vi "mitutoyo.vi"() -> ()   [LabVIEW 2015]
uses:
  <vilib>/Analysis/baseanly.llb/Mean (DBL).vi
  Global_mitu.vi
  <vilib>/Analysis/NI_AALBase.lvlib
panel:
  out "element":i32
  out "max value":dbl
  out "min value":dbl
  in  "DONE?":bool
  out "standard deviation":dbl format="%0.2f"
  out "mean":dbl format="%0.2f"
  out "Foil Name":string
  out "Output File path":path
  out "Result 9":bool
  out "Result 8":bool
  out "Result 7":bool
  out "Result 6":bool
  out "Result 5":bool
  out "Result 4":bool
  out "Result 3":bool
  out "Result 2":bool
  out "Result 1":bool
  in  "Open DataBase":bool
  out "9":bool
  out "8":bool
  out "7":bool
  out "6":bool
  out "5":bool
  out "4":bool
  out "3":bool
  out "2":bool
  out "1":bool
  in  "Table Control":string[][](table)
  in  "Stop\nMeasurement":bool
  # "Mitutoyo Honeycomb Measurements"
  # "Results"
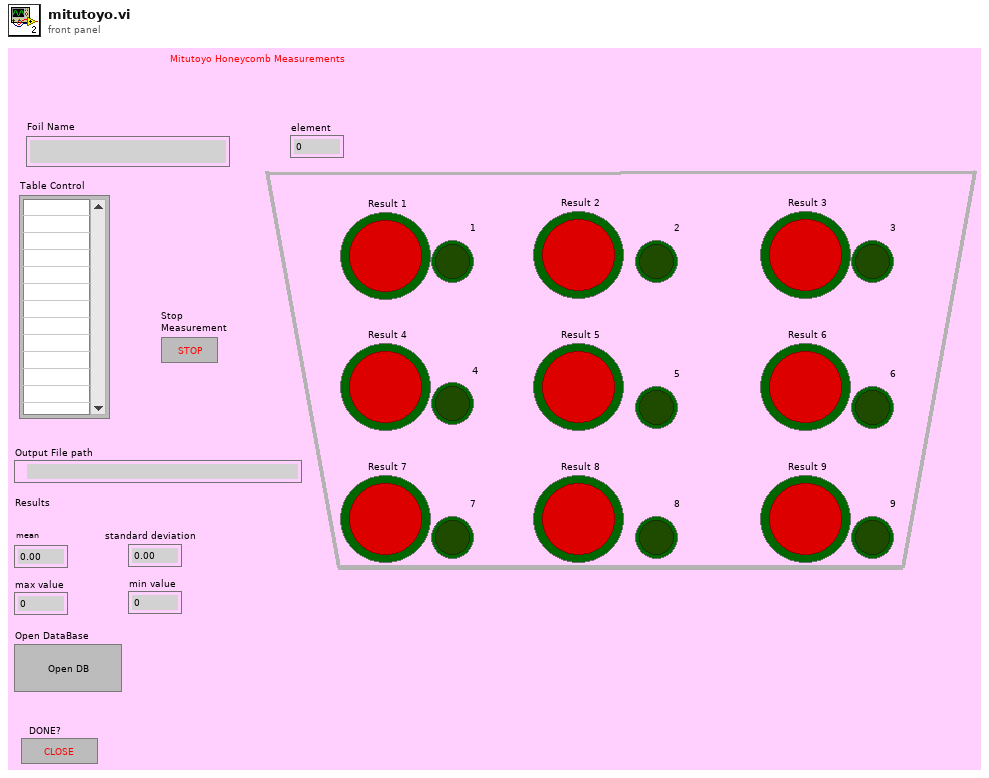
[diagram p1: front panel]
types:
  T1 = enum8{"Enabled", "Disabled", "Disabled and Grayed Out"}
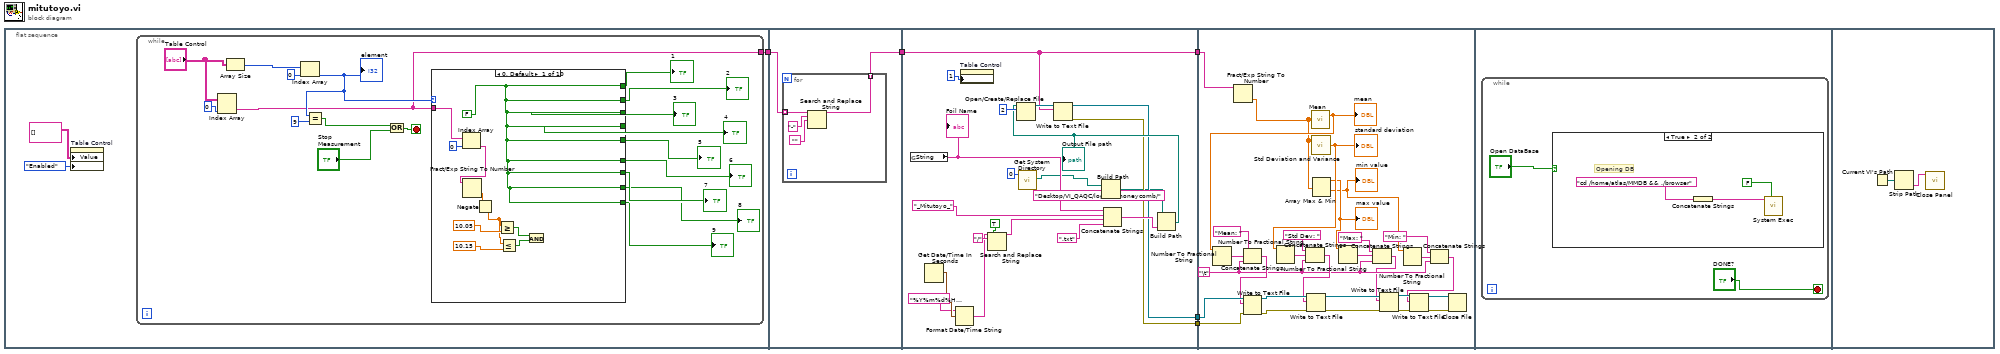
[diagram p0: block diagram]
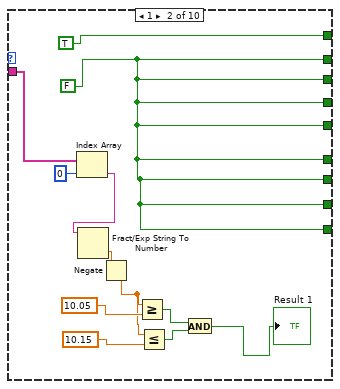
[diagram p2: hidden frame]
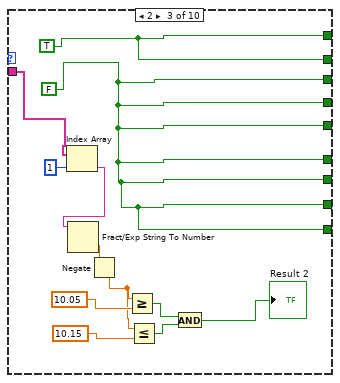
[diagram p3: hidden frame]
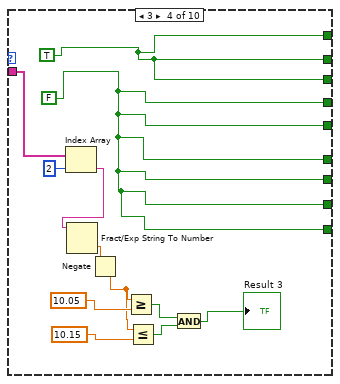
[diagram p4: hidden frame]
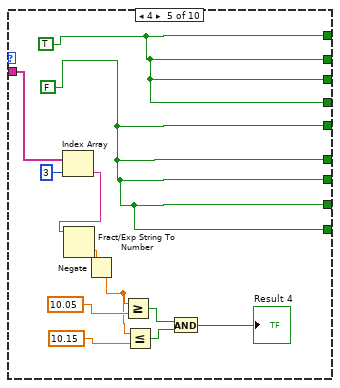
[diagram p5: hidden frame]
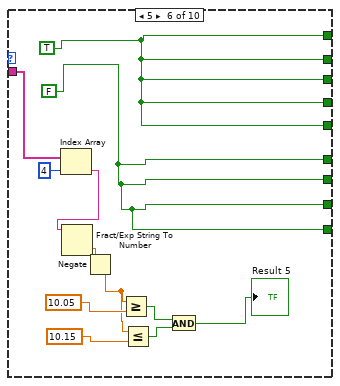
[diagram p6: hidden frame]
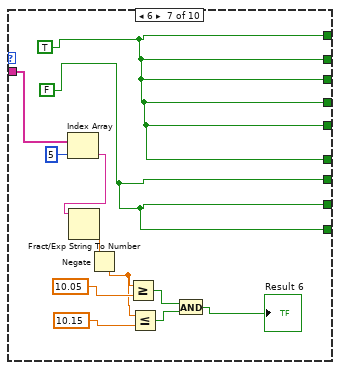
[diagram p7: hidden frame]
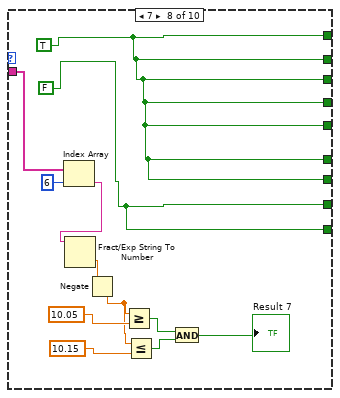
[diagram p8: hidden frame]
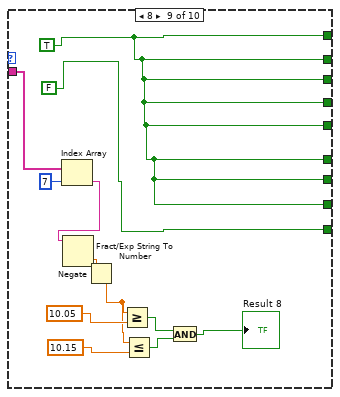
[diagram p9: hidden frame]
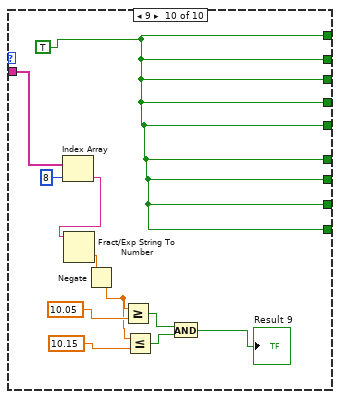
[diagram p10: hidden frame]
diagram:
  n1 = flat-sequence {
    tunnel: [w8] -> w2
    tunnel: w2 -> [w146]
    tunnel: [w145] -> w1
    tunnel: w1 -> [w151]
    tunnel: [w151] -> w5
    tunnel: [w160] -> w4
    tunnel: [w161] -> w3
    tunnel: w5 -> [w200]
    tunnel: w4 -> [w199]
    tunnel: w3 -> [w194]
    frame #0 {
      n2 = property on="Table Control" class="Tbl (strict)"("Value"=string[][] [] ("Table Control"), "DisabledEnum"=T1."Enabled" ("Disabled")) -> ()  [unwired: 2 in, 2 out]
      n3 = while {
        tunnel: [w10] -> w8
        stop <- w9 stop-if-true
        n4 = Index Array(array="Table Control", index (col)=0 ("index (row)")) -> (element=w10:string[])  [unwired: 1 in]
        n5 = Array Size(array="Table Control") -> (size(s)=w27:i32[])
        n6 = Index Array(array=w27, index=0) -> (element=w14:i32)
        "element" <- w14
        n7 = Equal?(x=w14, y=9) -> (x = y?=w11:bool)
        n8 = Or(x=w11, y="Stop\nMeasurement") -> (x .or. y?=w9:bool)
        n9 = case shown="0, Default" w14 {
          tunnel: [w37 TRUE w60 w73 w85 w97 w109 w121 w133 w144] -> w23
          tunnel: [w37 w48 w60 w73 w85 w97 w109 w121 w133 w144] -> w22
          tunnel: [w37 w48 w61 w73 w85 w97 w109 w121 w133 w144] -> w21
          tunnel: [w37 w48 w61 w72 w85 w97 w109 w121 w133 w144] -> w20
          tunnel: [w37 w48 w61 w72 w84 w97 w109 w121 w133 w144] -> w19
          tunnel: [w37 w48 w61 w72 w84 w96 w109 w121 w133 w144] -> w18
          tunnel: [w37 w48 w61 w72 w84 w96 w108 w121 w133 w144] -> w17
          tunnel: [w37 w48 w61 w72 w84 w96 w108 w120 w133 w144] -> w16
          tunnel: [w37 w48 w61 w72 w84 w96 w108 w120 FALSE w144] -> w15
          tunnel: w10 -> [w36 w40 w52 w64 w76 w88 w100 w112 w124 w136]
          frame 0, Default {
            w37 = FALSE
            n10 = Index Array(array=w36, index=0) -> (element=w34:string)
            n11 = Fract/Exp String To Number(string=w34) -> (number=w33:dbl)  [unwired: 3 in, 1 out]
            n12 = Negate(x=w33) -> (-x=w28:dbl)
            n13 = Greater Or Equal?(x=w28, y=10.05) -> (x >= y?=w32:bool)
            n14 = Less Or Equal?(x=w28, y=10.15) -> (x <= y?=w31:bool)
            n15 = And(x=w32, y=w31) -> ()  [unwired: 1 out]
          }
          frame 1 {
            w48 = FALSE
            n16 = Index Array(array=w40, index=0) -> (element=w41:string)
            n17 = Fract/Exp String To Number(string=w41) -> (number=w46:dbl)  [unwired: 3 in, 1 out]
            n18 = Negate(x=w46) -> (-x=w38:dbl)
            n19 = Greater Or Equal?(x=w38, y=10.05) -> (x >= y?=w45:bool)
            n20 = Less Or Equal?(x=w38, y=10.15) -> (x <= y?=w44:bool)
            n21 = And(x=w45, y=w44) -> (x .and. y?=→"Result 1":bool)
          }
          frame 2 {
            w61 = FALSE
            w60 = TRUE
            n22 = Index Array(array=w52, index=1) -> (element=w58:string)
            n23 = Fract/Exp String To Number(string=w58) -> (number=w57:dbl)  [unwired: 3 in, 1 out]
            n24 = Negate(x=w57) -> (-x=w50:dbl)
            n25 = Greater Or Equal?(x=w50, y=10.05) -> (x >= y?=w56:bool)
            n26 = Less Or Equal?(x=w50, y=10.15) -> (x <= y?=w55:bool)
            n27 = And(x=w56, y=w55) -> (x .and. y?=→"Result 2":bool)
          }
          frame 3 {
            w72 = FALSE
            w73 = TRUE
            n28 = Index Array(array=w64, index=2) -> (element=w70:string)
            n29 = Fract/Exp String To Number(string=w70) -> (number=w69:dbl)  [unwired: 3 in, 1 out]
            n30 = Negate(x=w69) -> (-x=w62:dbl)
            n31 = Greater Or Equal?(x=w62, y=10.05) -> (x >= y?=w68:bool)
            n32 = Less Or Equal?(x=w62, y=10.15) -> (x <= y?=w67:bool)
            n33 = And(x=w68, y=w67) -> (x .and. y?=→"Result 3":bool)
          }
          frame 4 {
            w84 = FALSE
            w85 = TRUE
            n34 = Index Array(array=w76, index=3) -> (element=w82:string)
            n35 = Fract/Exp String To Number(string=w82) -> (number=w81:dbl)  [unwired: 3 in, 1 out]
            n36 = Negate(x=w81) -> (-x=w74:dbl)
            n37 = Greater Or Equal?(x=w74, y=10.05) -> (x >= y?=w80:bool)
            n38 = Less Or Equal?(x=w74, y=10.15) -> (x <= y?=w79:bool)
            n39 = And(x=w80, y=w79) -> (x .and. y?=→"Result 4":bool)
          }
          frame 5 {
            w96 = FALSE
            w97 = TRUE
            n40 = Index Array(array=w88, index=4) -> (element=w94:string)
            n41 = Fract/Exp String To Number(string=w94) -> (number=w93:dbl)  [unwired: 3 in, 1 out]
            n42 = Negate(x=w93) -> (-x=w86:dbl)
            n43 = Greater Or Equal?(x=w86, y=10.05) -> (x >= y?=w92:bool)
            n44 = Less Or Equal?(x=w86, y=10.15) -> (x <= y?=w91:bool)
            n45 = And(x=w92, y=w91) -> (x .and. y?=→"Result 5":bool)
          }
          frame 6 {
            w108 = FALSE
            w109 = TRUE
            n46 = Index Array(array=w100, index=5) -> (element=w102:string)
            n47 = Fract/Exp String To Number(string=w102) -> (number=w103:dbl)  [unwired: 3 in, 1 out]
            n48 = Negate(x=w103) -> (-x=w98:dbl)
            n49 = Greater Or Equal?(x=w98, y=10.05) -> (x >= y?=w104:bool)
            n50 = Less Or Equal?(x=w98, y=10.15) -> (x <= y?=w105:bool)
            n51 = And(x=w104, y=w105) -> (x .and. y?=→"Result 6":bool)
          }
          frame 7 {
            w120 = FALSE
            w121 = TRUE
            n52 = Index Array(array=w112, index=6) -> (element=w118:string)
            n53 = Fract/Exp String To Number(string=w118) -> (number=w117:dbl)  [unwired: 3 in, 1 out]
            n54 = Negate(x=w117) -> (-x=w110:dbl)
            n55 = Greater Or Equal?(x=w110, y=10.05) -> (x >= y?=w116:bool)
            n56 = Less Or Equal?(x=w110, y=10.15) -> (x <= y?=w115:bool)
            n57 = And(x=w116, y=w115) -> (x .and. y?=→"Result 7":bool)
          }
          frame 8 {
            w133 = TRUE
            n58 = Index Array(array=w124, index=7) -> (element=w130:string)
            n59 = Fract/Exp String To Number(string=w130) -> (number=w129:dbl)  [unwired: 3 in, 1 out]
            n60 = Negate(x=w129) -> (-x=w122:dbl)
            n61 = Greater Or Equal?(x=w122, y=10.05) -> (x >= y?=w128:bool)
            n62 = Less Or Equal?(x=w122, y=10.15) -> (x <= y?=w127:bool)
            n63 = And(x=w128, y=w127) -> (x .and. y?=→"Result 8":bool)
          }
          frame 9 {
            w144 = TRUE
            n64 = Index Array(array=w136, index=8) -> (element=w142:string)
            n65 = Fract/Exp String To Number(string=w142) -> (number=w141:dbl)  [unwired: 3 in, 1 out]
            n66 = Negate(x=w141) -> (-x=w134:dbl)
            n67 = Greater Or Equal?(x=w134, y=10.05) -> (x >= y?=w140:bool)
            n68 = Less Or Equal?(x=w134, y=10.15) -> (x <= y?=w139:bool)
            n69 = And(x=w140, y=w139) -> (x .and. y?=→"Result 9":bool)
          }
        }
        "1" <- w23
        "2" <- w22
        "3" <- w21
        "4" <- w20
        "5" <- w19
        "6" <- w18
        "7" <- w17
        "8" <- w16
        "9" <- w15
      }
    }
    frame #1 {
      n70 = for {
        tunnel: w146 -> [w150] mode=indexing
        tunnel: [w147] -> w145 mode=indexing
        n71 = Search and Replace String(input string=w150, search string="-", replace string="") -> (result string=w147:string)  [unwired: 5 in, 3 out]
      }
    }
    frame #2 {
      n72 = global read "Global_mitu.vi" "String"() -> (w168:string)
      "Foil Name" <- w168
      n73 = Get Date/Time In Seconds() -> (seconds since 1Jan1904=w159:timestamp)
      n74 = Format Date/Time String(time format string (%c)="%Y%m%d%H%M", seconds (now)=w159) -> (date/time string=w157:string)  [unwired: 1 in]
      n75 = property on="Table Control" class="Tbl (strict)"("DisabledEnum"=1) -> ()  [unwired: 2 in, 2 out]
      n76 = Search and Replace String(replace all?=TRUE ("replace all? (F)"), input string=w157, search string="/") -> (result string=w166:string)  [unwired: 5 in, 3 out]
      n77 = call <vilib>:"Get System Directory.vi"("system directory type"=0) -> ("system directory"=w154:path)  [unwired: 10 in]
      n78 = Build Path(base path=w154, name or relative path="Desktop/VI_QAQC/logfiles/honeycomb/") -> (appended path=w153:path)
      n79 = Concatenate Strings(w168, "_Mitutoyo_", w166, ".txt") -> (w164:string)
      n80 = Build Path(base path=w153, name or relative path=w164) -> (appended path=w169:path)
      "Output File path" <- w169
      n81 = Open/Create/Replace File(file path (use dialog)=w169, operation (0:open)=2) -> (refnum out=w170:refnum<file>)  [unwired: 4 in, 2 out]
      n82 = Write to Text File(file (use dialog)=w170, text=w151) -> (refnum out=w160:refnum<file>, error out=w161:errorcluster)  [unwired: 2 in, 1 out]
    }
    frame #3 {
      w183 = "\t"
      n83 = Fract/Exp String To Number(string=w200) -> (number=w191:dbl[])  [unwired: 3 in, 1 out]
      n84 = call-poly <vilib>:"Mean.vi"("X"=w191) -> ("mean"=w198:dbl)  [unwired: 1 out]
      "mean" <- w198
      n85 = Number To Fractional String(number=w198) -> (F-format string=w193:string)  [unwired: 3 in]
      n86 = Concatenate Strings("Mean: ", w193, w183) -> (w192:string)
      n87 = Write to Text File(file (use dialog)=w199, text=w192, error in=w194) -> (refnum out=w197:refnum<file>, error out=w195:errorcluster)  [unwired: 1 in, 1 out]
      n88 = call <vilib>:"Std Deviation and Variance.vi"("X"=w191) -> ("standard deviation"=w196:dbl)  [unwired: 1 in, 2 out]
      "standard deviation" <- w196
      n89 = Number To Fractional String(number=w196) -> (F-format string=w190:string)  [unwired: 3 in]
      n90 = Concatenate Strings("Std Dev: ", w190, w183) -> (w189:string)
      n91 = Write to Text File(file (use dialog)=w197, text=w189, error in=w195) -> (refnum out=w188:refnum<file>, error out=w180:errorcluster)  [unwired: 1 in, 1 out]
      n92 = Array Max & Min(array=w191) -> (max value=w173:dbl, min value=w172:dbl)  [unwired: 2 out]
      "min value" <- w172
      "max value" <- w173
      n93 = Number To Fractional String(number=w173) -> (F-format string=w185:string)  [unwired: 3 in]
      n94 = Concatenate Strings("Max: ", w185, w183) -> (w181:string)
      n95 = Write to Text File(file (use dialog)=w188, text=w181, error in=w180) -> (refnum out=w187:refnum<file>, error out=w179:errorcluster)  [unwired: 1 in, 1 out]
      n96 = Number To Fractional String(number=w172) -> (F-format string=w184:string)  [unwired: 3 in]
      n97 = Concatenate Strings("Min: ", w184, w183) -> (w182:string)
      n98 = Write to Text File(file (use dialog)=w187, text=w182, error in=w179) -> (refnum out=w186:refnum<file>, error out=w178:errorcluster)  [unwired: 1 in, 1 out]
      n99 = Close File(refnum=w186, error in=w178) -> ()  [unwired: 2 out]
    }
    frame #4 {
      n100 = while {
        stop <- "DONE?" stop-if-true
        n101 = case shown="True" "Open DataBase" {
          frame False {
          }
          frame True {
            # "Opening DB"
            n102 = Concatenate Strings("cd /home/atlas/MMDB && ./browser") -> (w204:string)
            n103 = call <vilib>:"System Exec.vi"("wait until completion? (T)"=FALSE, "command line"=w204) -> ()  [unwired: 6 in, 4 out]
          }
        }
      }
    }
    frame #5 {
      n104 = Current VI's Path() -> (path=w207:path)
      n105 = Strip Path(path=w207) -> (name=w206:string)  [unwired: 1 out]
      n106 = call <vilib>:"Close Panel.vi"("VI name"=w206) -> ()  [unwired: 10 in, 1 out]
    }
  }
